vi "Clear Interlock Alarm.vi"(8 "error in":errorcluster, 11 "5745A in":refnum<class "5745A.lvclass">) -> (0 "error out":errorcluster, 3 "5745A out":refnum<class "5745A.lvclass">)   [LabVIEW 2018, in "5745A.lvlib" / "5745A.lvclass"]
uses:
  5745A.lvclass
  builds/Power_Supply.lvlibp/Power Supply.lvclass
  C:/Users/Ron.Dexter.LUMINARTECH/Desktop/builds/Power_Supply.lvlibp/Power Supply.lvclass
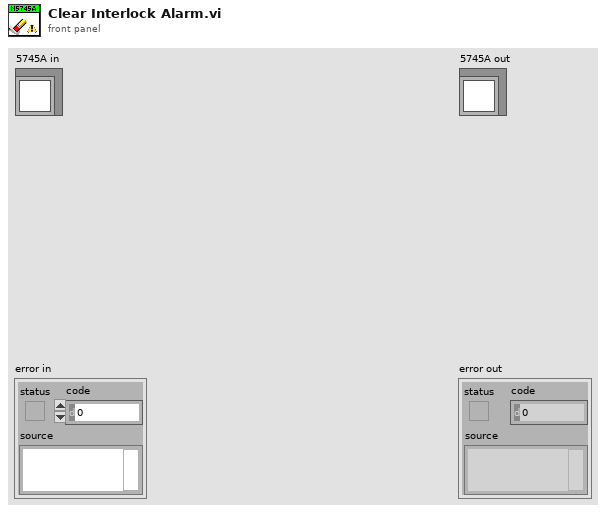
[diagram p1: front panel]
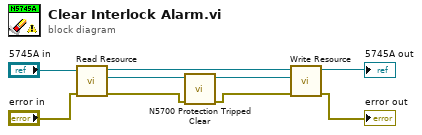
[diagram p0: block diagram]
diagram:
  n1 = call "Read Resource.vi"("error in"="error in", "Power Supply in"="5745A in") -> ("error out"=w2:errorcluster, "Resource"=w4:refnum<visa-resource-name>, "Power Supply out"=w7:refnum<class "5745A.lvclass">)  [unwired: 7 in]
  n2 = call <instrlib>:"N5700 Protection Tripped Clear.vi"("error"=w2, "VISA"=w4) -> ("error out"=w1:errorcluster, "VISA out"=w3:refnum<visa-resource-name>)  [unwired: 5 in]
  n3 = call "Write Resource.vi"("error in"=w1, "Resource"=w3, "Power Supply in"=w7) -> ("error out"=→"error out":errorcluster, "Power Supply out"=→"5745A out":refnum<class "5745A.lvclass">)  [unwired: 7 in]
